vi "Read piece.vi"(8 "error in (no error)":errorcluster, 10 "Square":T1={"File"=enum."a", "Rank"=enum."4"}, 11 "Position in":refnum<class "Position.lvclass">) -> (0 "error out":errorcluster, 2 "Piece":refnum<class "Piece.lvclass">, 3 "Position out":refnum<class "Position.lvclass">)   [LabVIEW 2016, in "Chesslib.lvlib" / "Position.lvclass"]
uses:
  Position.lvclass
  typedef/Square.ctl
  typedef/File.ctl
  typedef/Rank.ctl
  Pieces/Piece/Piece.lvclass
  Position.lvclass/Position.ctl
  Board/Board.lvclass
  Chesslib.lvlib
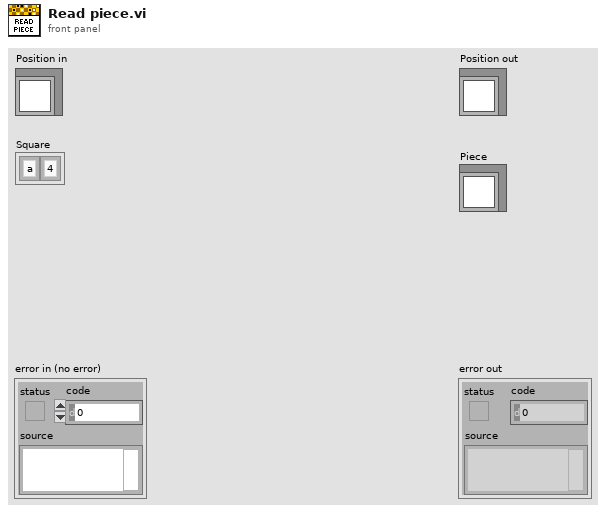
[diagram p1: front panel]
types:
  T1 = typedef "Chesslib.lvlib/Square.ctl" = cluster{"File":T2, "Rank":T3}
  T2 = typedef "Chesslib.lvlib/File.ctl" = enum8{"a", "b", "c", "d", "e", "f", "g", "h"}
  T3 = typedef "Chesslib.lvlib/Rank.ctl" = enum8{"1", "2", "3", "4", "5", "6", "7", "8"}
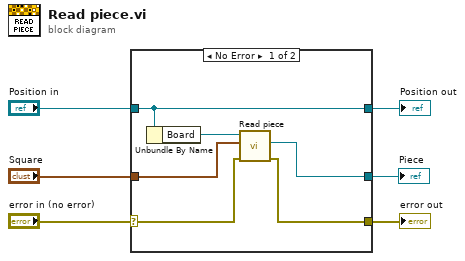
[diagram p0: block diagram]
diagram:
  n1 = case shown="No Error" "error in (no error)" {
    selector: "error in (no error)" -> [w9 w14]
    tunnel: [w8 w14] -> w5
    tunnel: [w12 w13] -> w3
    tunnel: "Position in" -> [w12 w13]
    tunnel: "Square" -> [w10 _]
    tunnel: [w7 _] -> w1
    frame No Error {
      n2 = Unbundle By Name(w12) -> ("Board"=w11:refnum<class "Board.lvclass">)
      n3 = call "Read piece.vi"("error in (no error)"=w9, "Square"=w10, "Board in"=w11) -> ("error out"=w8:errorcluster, "Piece"=w7:refnum<class "Piece.lvclass">)  [unwired: 6 in, 1 out]
    }
    frame Error {
    }
  }
  "error out" <- w5
  "Position out" <- w3
  "Piece" <- w1
